vi "splitarray.vi"() -> ()   [LabVIEW 2015]
uses:
  <vilib>/Analysis/Matrix/Datatypes/RealMatrix.ctl
  <vilib>/Analysis/Matrix/NI_Matrix.lvlib
panel:
  out "Array 3":dbl[][](array[numeric])
  out "columns":i32
  out "rows":i32
  in  "Real Matrix":T1
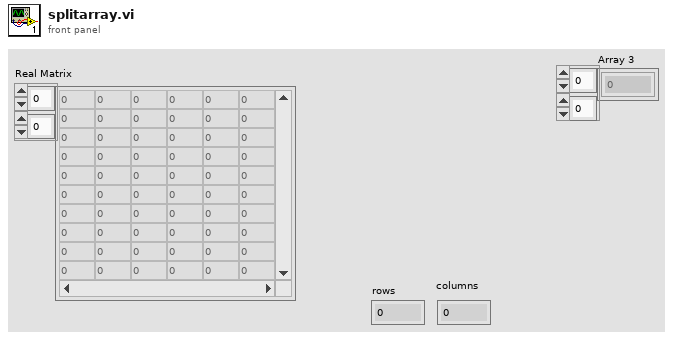
[diagram p1: front panel]
types:
  T1 = typedef "NI_Matrix.lvlib/RealMatrix.ctl" = dbl[][]
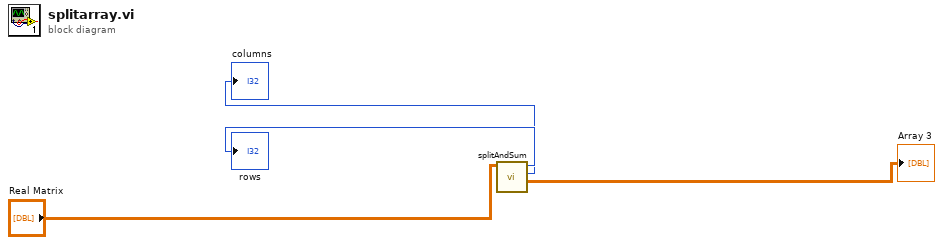
[diagram p0: block diagram]
diagram:
  n1 = call "splitAndSum.vi"("Real Matrix"="Real Matrix") -> ("Array"=→"Array 3":dbl[][], "columns"=→"columns":i32, "rows"=→"rows":i32)  [unwired: 8 in]
